vi "Configure Frequency Counter.vi"(0 "VISA resource name":refnum<visa-resource-name>, 5 "Marker Set (0:Marker 1)":i32(ring) items=["Marker 1", "Marker 2", "Marker 3", "Marker 4", "Marker 5", "Marker 6", "Marker 7", "Marker 8", "Marker 9", "Marker 10", "None"], 7 "Frequency Counter (1:On)":i32(ring)=1 items=["Off", "On"], 9 "Gate Time (0.01s)":dbl=0.01 min=0.0001 max=1.0, 11 "error in (no error)":errorcluster) -> (4 "VISA resource name out":refnum<visa-resource-name>, 15 "error out":errorcluster)   [LabVIEW 2020, in "Anritsu Signal Analyzer Series.lvlib"]
doc: "Configures the frequency counter settings of the spectrum analyzer."
uses:
  Anritsu Signal Analyzer Series.lvlib
panel:
  # "s"
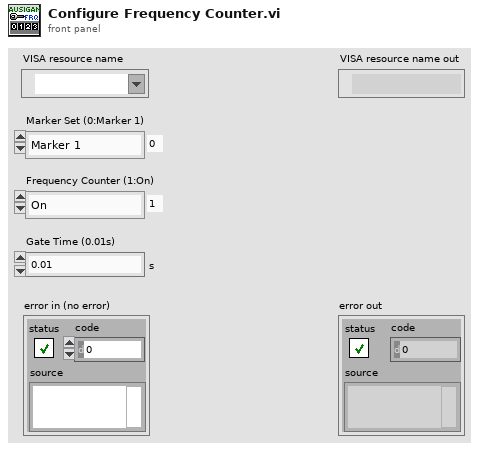
[diagram p1: front panel]
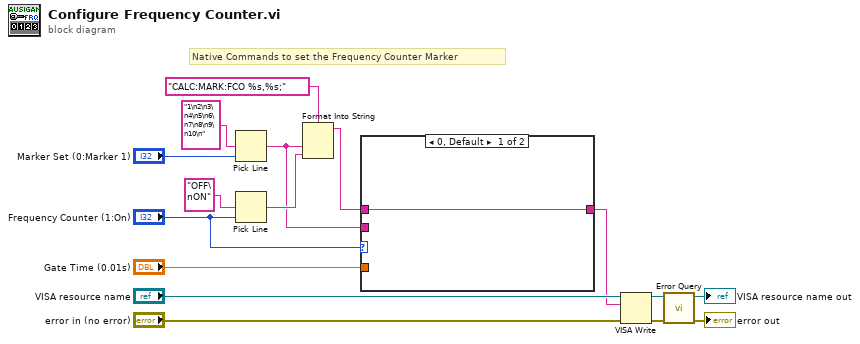
[diagram p0: block diagram]
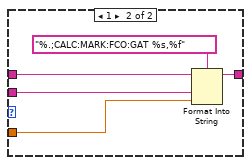
[diagram p2: hidden frame]
diagram:
  # "Native Commands to set the Frequency Counter Marker"
  n1 = Pick Line(multi-line string="1\n2\n3\n4\n5\n6\n7\n8\n9\n10\n" ("文字列"), line index="Marker Set (0:Marker 1)") -> (output string=w3:string)  [unwired: 1 in]
  n2 = Pick Line(multi-line string="OFF\nON" ("複数行文字列"), line index="Frequency Counter (1:On)") -> (output string=w5:string)  [unwired: 1 in]
  n3 = Format Into String(format string="CALC:MARK:FCO %s,%s;" ("_CommandSet"), w3, w5) -> (resulting string=w8:string)  [unwired: 2 in, 1 out]
  n4 = case shown="0, Default" "Frequency Counter (1:On)" {
    tunnel: "Gate Time (0.01s)" -> [_ w22]
    tunnel: w3 -> [_ w21]
    tunnel: w8 -> [w17 w20]
    tunnel: [w17 w18] -> w7
    frame 0, Default {
    }
    frame 1 {
      n5 = Format Into String(format string="%.;CALC:MARK:FCO:GAT %s,%f" ("_Command Set"), initial string=w20, w21, w22) -> (resulting string=w18:string)  [unwired: 1 in, 1 out]
    }
  }
  n6 = VISA Write(VISA resource name="VISA resource name", write buffer=w7, error in (no error)="error in (no error)") -> (VISA resource name out=w12:refnum<visa-resource-name>, error out=w13:errorcluster)  [unwired: 1 out]
  n7 = call "Error Query.vi"("error in (no error)"=w13, "VISA resource name"=w12) -> ("error out"=→"error out":errorcluster, "VISA resource name out"=→"VISA resource name out":refnum<visa-resource-name>)  [unwired: 6 in, 2 out]
